vi "Edit-dialog.vi"(8 "error in (no error)":errorcluster, 11 "Action in":refnum<class "Wait.lvclass">) -> (0 "error out":errorcluster, 3 "Action out":refnum<class "Wait.lvclass">)   [LabVIEW 2013, in "PowderDeposition.lvlib" / "Wait.lvclass"]
uses:
  Wait.lvclass
  Wait.lvclass/Wait.ctl
panel:
  in  "Cancel":bool
  in  "OK":bool
  in  "Edit dialog":cluster{"Duration [s]":dbl}
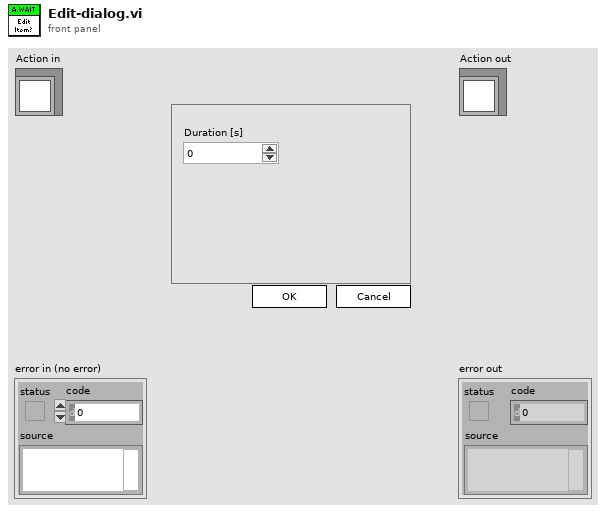
[diagram p1: front panel]
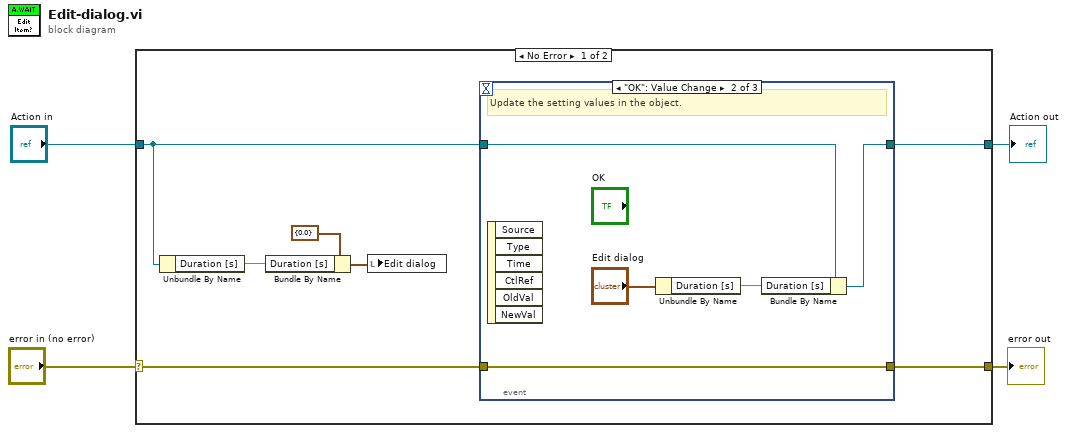
[diagram p0: block diagram]
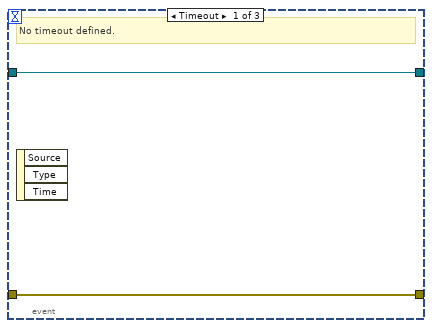
[diagram p2: hidden frame]
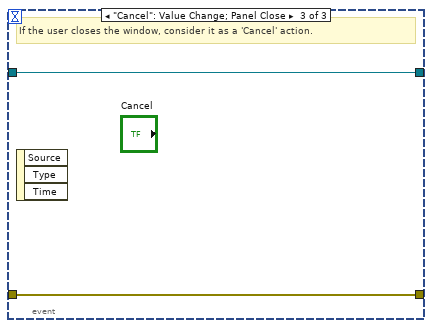
[diagram p3: hidden frame]
diagram:
  n1 = case shown="No Error" "error in (no error)" {
    selector: "error in (no error)" -> [w10 w22]
    tunnel: [w9 w22] -> w3
    tunnel: [w11 w21] -> w1
    tunnel: "Action in" -> [w6 w21]
    frame No Error {
      n2 = Unbundle By Name(w6) -> ("Duration [s]"=w8:dbl)
      n3 = Bundle By Name(cluster=cluster{"Duration [s]":dbl} {"Duration [s]"=0.0} ("Edit dialog 2"), "Duration [s]"=w8) -> (w5:cluster{"Duration [s]":dbl})
      n4 = local write "Edit dialog"(w5) -> ()
      n5 = event shown="[1] \"OK\": Value Change" {
        selector: _ -> [_ _ _]
        dyn-events: _ -> [_ _ _]
        timeout: _ -> [_ _ _]
        tunnel: w6 -> [w13 w17 w20]
        tunnel: [w13 w16 w20] -> w11
        tunnel: w10 -> [w12 w18 w19]
        tunnel: [w12 w18 w19] -> w9
        event Timeout {
          # "No timeout defined."
          n6 = event-data() -> ()  [unwired: 1 in, 3 out]
        }
        event "OK": Value Change {
          # "Update the setting values in the object."
          n7 = event-data() -> ()  [unwired: 1 in, 6 out]
          n8 = Unbundle By Name("Edit dialog") -> ("Duration [s]"=w14:dbl)
          n9 = Bundle By Name(cluster=w17, "Duration [s]"=w14) -> (w16:refnum<class "Wait.lvclass">)
        }
        event "Cancel": Value Change; Panel Close {
          # "If the user closes the window, consider it as a 'Cancel' action."
          n10 = event-data() -> ()  [unwired: 1 in, 3 out]
        }
      }
    }
    frame Error {
    }
  }
  "error out" <- w3
  "Action out" <- w1
